vi "decoder.vi"(11 "Read Buffer":string) -> (3 "string":string)   [LabVIEW 2020]
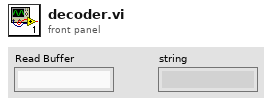
[diagram p1: front panel]
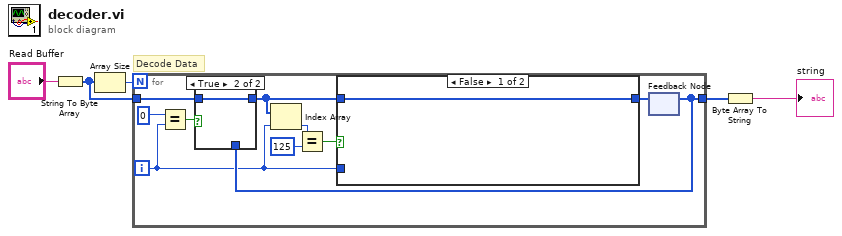
[diagram p0: block diagram]
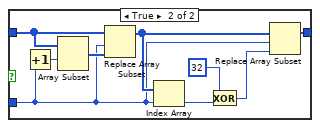
[diagram p3: hidden frame]
diagram:
  # "Decode Data"
  n1 = String To Byte Array(string="Read Buffer") -> (unsigned byte array=w1:u8[])
  n2 = Array Size(array=w1) -> (size(s)=w2:i32)
  n3 = for {
    N: w2 -> [_]
    tunnel: w1 -> [w10]
    tunnel: [w9] -> w3
    i -> [w8]
    n4 = Equal?(x=0 ("y"), y=w8) -> (x = y?=w12:bool)
    n5 = feedback #1() -> (w9:u8[])  [unwired: 1 in]
    n6 = case shown="True" w12 {
      tunnel: [w16 w17] -> w11
      tunnel: w10 -> [_ w17]
      tunnel: w9 -> [w16 _]
      frame False {
      }
      frame True {
      }
    }
    n7 = Index Array(array=w11, index=w8) -> (element=w13:u8)
    n8 = Equal?(x=w13, y=u8 125) -> (x = y?=w14:bool)
    n9 = case shown="False" w14 {
      tunnel: w11 -> [w18 w25]
      tunnel: w8 -> [_ w23]
      tunnel: [w18 w26] -> w6
      frame False {
      }
      frame True {
        n10 = Increment(x=w23) -> (x+1=w22:i32)
        n11 = Array Subset(array=w25, index=w22) -> (w27:u8[])  [unwired: 1 in]
        n12 = Replace Array Subset(array=w25, new element=w27, index=w23) -> (w24:u8[])
        n13 = Index Array(array=w24, index=w23) -> (element=w21:u8)
        n14 = Exclusive Or(1:w21, 2:u8 32 ("y")) -> (0:w19:u8)
        n15 = Replace Array Subset(array=w24, new element=w19, index=w23) -> (w26:u8[])
      }
    }
    n16 = feedback-in #1(w6) -> ()
  }
  n17 = Byte Array To String(unsigned byte array=w3) -> (string=→"string":string)
